vi "WriteDataSources.vi"(8 "error in (no error)":errorcluster, 11 "body":u8[](array[numeric])) -> (0 "error out":errorcluster)   [LabVIEW 2017, in "ServerComm.lvlib"]
uses:
  <vilib>/addons/InsightCM/Devices/Shared/Common/ServerComm/ServerComm.lvlib
  <vilib>/addons/InsightCM/MessageBus/Base/controls/DataSource.ctl
  <vilib>/addons/InsightCM/MessageBus/Base/controls/KeyValuePair.ctl
  <vilib>/addons/InsightCM/Utilities/GlobalConfiguration/GlobalConfiguration.lvlib
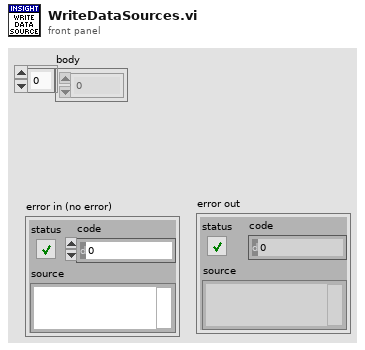
[diagram p1: front panel]
types:
  T1 = cluster{"DataSourceId":string, "Filename":string, "Contents":string}[]
  T2 = typedef "DataSource.ctl" = cluster{"Id":string, "Type":string, "Name":string, "MeasType":string, "Properties":T3[]}
  T3 = typedef "KeyValuePair.ctl" = cluster{"Key":string, "Value":string}
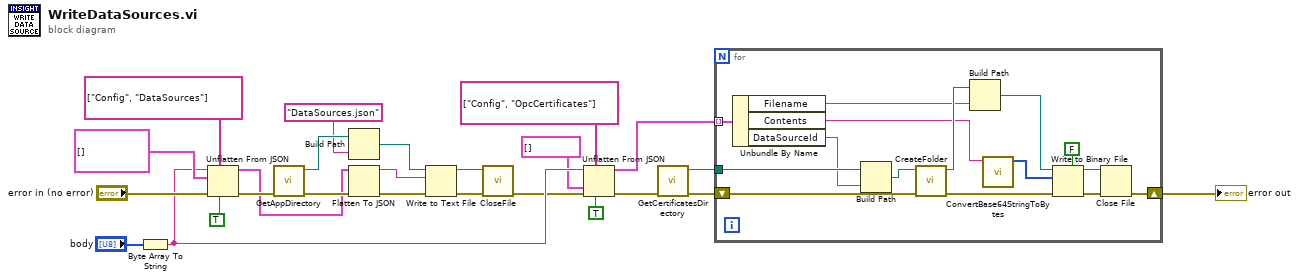
[diagram p0: block diagram]
diagram:
  n1 = Byte Array To String(unsigned byte array="body") -> (string=w8:string)
  n2 = Unflatten From JSON(path=string[] ["Config", "DataSources"], JSON string=w8, type and defaults=T2[] [] ("data sources"), default null elements? (F)=TRUE, error in (no error)="error in (no error)") -> (value=w11:T2[], error out=w14:errorcluster)  [unwired: 2 in]
  n3 = call <vilib>:"GetAppDirectory.vi"("error in (no error)"=w14) -> ("error out"=w23:errorcluster, "application directory"=w25:path)  [unwired: 9 in]
  n4 = Build Path(base path=w25, name or relative path="DataSources.json") -> (appended path=w21:path)
  n5 = Flatten To JSON(anything=w11, error in (no error)=w23) -> (JSON string=w20:string, 11:w22:errorcluster)  [unwired: 1 in]
  n6 = Write to Text File(file (use dialog)=w21, text=w20, error in=w22) -> (refnum out=w19:refnum<file>, error out=w18:errorcluster)  [unwired: 1 in, 1 out]
  n7 = call <vilib>:"CloseFile.vi"("error in (no error)"=w18, "file reference"=w19) -> ("error out"=w6:errorcluster)  [unwired: 9 in]
  n8 = Unflatten From JSON(path=string[] ["Config", "OpcCertificates"], JSON string=w8, type and defaults=T1 [], default null elements? (F)=TRUE, error in (no error)=w6) -> (value=w4:T1, error out=w5:errorcluster)  [unwired: 2 in]
  n9 = call <vilib>:"GetCertificatesDirectory.vi"("error in (no error)"=w5) -> ("error out"=w3:errorcluster, "application directory"=w2:path)  [unwired: 9 in]
  n10 = for {
    tunnel: w4 -> [w40] mode=indexing
    tunnel: w2 -> [w39]
    shift-right: [w26] -> w1
    shift-left: w3 -> [w36]
    n11 = Unbundle By Name(w40) -> ("Filename"=w32:string, "Contents"=w31:string, "DataSourceId"=w38:string)
    n12 = Build Path(base path=w39, name or relative path=w38) -> (appended path=w37:path)
    n13 = call <vilib>:"CreateFolder.vi"("error in (no error)"=w36, "folder"=w37) -> ("error out"=w34:errorcluster, "folder out"=w35:path)  [unwired: 8 in]
    n14 = Build Path(base path=w35, name or relative path=w32) -> (appended path=w33:path)
    n15 = call <vilib>:"ConvertBase64StringToBytes.vi"("Base64 string"=w31) -> ("U8 array"=w30:u8[])  [unwired: 9 in, 1 out]
    n16 = Write to Binary File(file (use dialog)=w33, data=w30, error in=w34, 5:FALSE ("prepend array or string size? (T)")) -> (refnum out=w28:refnum<file>, error out=w27:errorcluster)  [unwired: 2 in, 1 out]
    n17 = Close File(refnum=w28, error in=w27) -> (error out=w26:errorcluster)  [unwired: 1 out]
  }
  "error out" <- w1
